vi "FPGA channel logic.vi"(2 "Pulse divide":u32=1 min=1 step=1, 3 "Accumulator in":u32, 4 "Channel ON at tick":u32, 5 "Pulse width (ticks)":u32, 6 "Current tick number":i32, 7 "Channel enabled?":bool) -> (0 "Accumulator out":u32, 1 "Channel ON/OFF":bool)   [LabVIEW 2013]
doc: "This SubVI implements the logic that controls whether an output channel should be HIGH or LOW.\n\nPulse division is implemented. The default pulse division value is 1, which makes the channel logic run on every cycle. If the pulse division is 2, the channel logic will run on every other cycle. If 5, the channel logic will run on every 5th cycle."
panel:
  # "FPGA channel logic"
  # "Generates signals to implement a rising-edge trigger\npulse for a single channel."
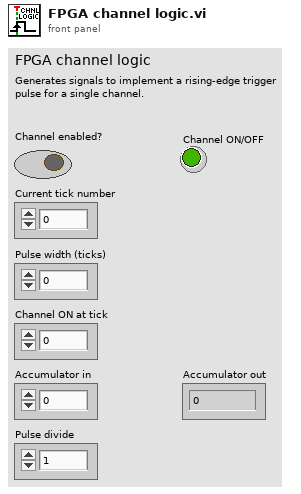
[diagram p1: front panel]
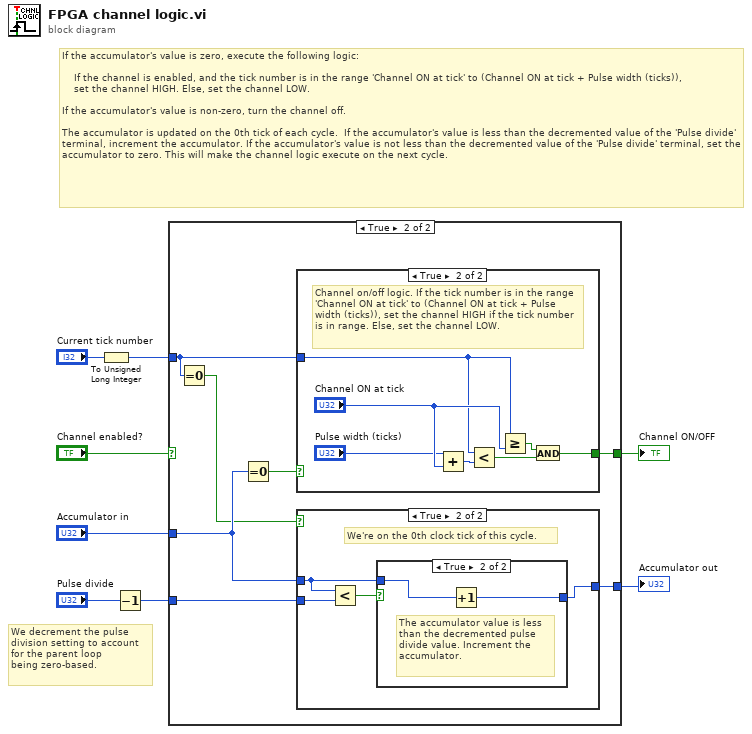
[diagram p0: block diagram]
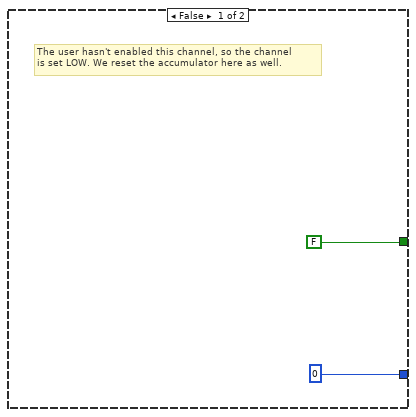
[diagram p2: hidden frame]
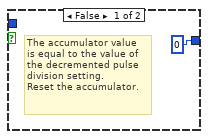
[diagram p4: hidden frame]
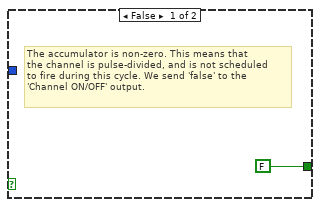
[diagram p5: hidden frame]
diagram:
  # "We decrement the pulse\ndivision setting to account\nfor the parent loop\nbeing zero-based."
  # "If the accumulator's value is zero, execute the following logic:\n\n    If the channel is enabled, and the tick number is in the range 'Channel ON at tick' to (Channel ON at tick + Pulse width (ticks)), \n    set the channel HIGH. Else, set the channel LOW.\n\nIf the accumulator's value is non-zero, turn the channel off.\n\nThe accumulator is updated on the 0th tick of each cycle.  If the accumulator's value is less than the decremented value of the 'Pulse divide' terminal, increment the accumulator. If the accumulator's value is not less than the decremented value of the 'Pulse divide' terminal, set the accumulator to zero. This will make the channel logic execute on the next cycle."
  n1 = To Unsigned Long Integer(number="Current tick number") -> (unsigned 32bit integer=w3:u32)
  n2 = Decrement(x="Pulse divide") -> (x-1=w1:u32)
  n3 = case shown="True" "Channel enabled?" {
    tunnel: [FALSE w17] -> w8
    tunnel: "Accumulator in" -> [_ w14]
    tunnel: [u32 0 ("Accumulator in") w13] -> w5
    tunnel: w1 -> [_ w15]
    tunnel: w3 -> [_ w12]
    frame False {
      # "The user hasn't enabled this channel, so the channel \nis set LOW. We reset the accumulator here as well."
    }
    frame True {
      n4 = Equal To 0?(x=w12) -> (x = 0?=w11:bool)
      n5 = Equal To 0?(x=w14) -> (x = 0?=w16:bool)
      n6 = case shown="True" w16 {
        tunnel: [FALSE w28] -> w17
        tunnel: w12 -> [_ w27]
        frame False {
          # "The accumulator is non-zero. This means that \nthe channel is pulse-divided, and is not scheduled\nto fire during this cycle. We send 'false' to the\n'Channel ON/OFF' output."
        }
        frame True {
          # "Channel on/off logic. If the tick number is in the range 'Channel ON at tick' to (Channel ON at tick + Pulse width (ticks)), set the channel HIGH if the tick number is in range. Else, set the channel LOW."
          n7 = Add(x="Pulse width (ticks)", y="Channel ON at tick") -> (x+y=w32:u32)
          n8 = Less?(x=w27, y=w32) -> (x < y?=w33:bool)
          n9 = Greater Or Equal?(x=w27, y="Channel ON at tick") -> (x >= y?=w31:bool)
          n10 = And(x=w31, y=w33) -> (x .and. y?=w28:bool)
        }
      }
      n11 = case shown="True" w11 {
        tunnel: w15 -> [_ w22]
        tunnel: w14 -> [w18 w20]
        tunnel: [w18 w19] -> w13
        frame False {
          # "We're not on the 0th clock tick of this cycle,\nso don't update the value of the accumulator."
        }
        frame True {
          # "We're on the 0th clock tick of this cycle."
          n12 = Less?(x=w20, y=w22) -> (x < y?=w21:bool)
          n13 = case shown="True" w21 {
            tunnel: w20 -> [_ w25]
            tunnel: [u32 0 ("Accumulator in") w24] -> w19
            frame False {
              # "The accumulator value\nis equal to the value of \nthe decremented pulse division setting.\nReset the accumulator."
            }
            frame True {
              # "The accumulator value is less\nthan the decremented pulse\ndivide value. Increment the\naccumulator."
              n14 = Increment(x=w25) -> (x+1=w24:u32)
            }
          }
        }
      }
    }
  }
  "Channel ON/OFF" <- w8
  "Accumulator out" <- w5
